vi "Write to Module.vi"(8 "error in (no error)":errorcluster, 9 "Data":u16, 10 "Module":enum16{"LAI", "LDO", "Control"}(ring), 11 "Modbus in":refnum<class "Modbus.lvclass">) -> (0 "error out":errorcluster, 3 "Modbus out":refnum<class "Modbus.lvclass">)   [LabVIEW 2020, in "Modbus.lvlib" / "Modbus.lvclass"]
uses:
  Modbus.lvclass
  Modbus.lvclass/Modbus.ctl
  <vilib>/NI Modbus.llb/MB Serial Master Query Write Multiple Registers (poly).vi
panel:
  in  "Register":u16
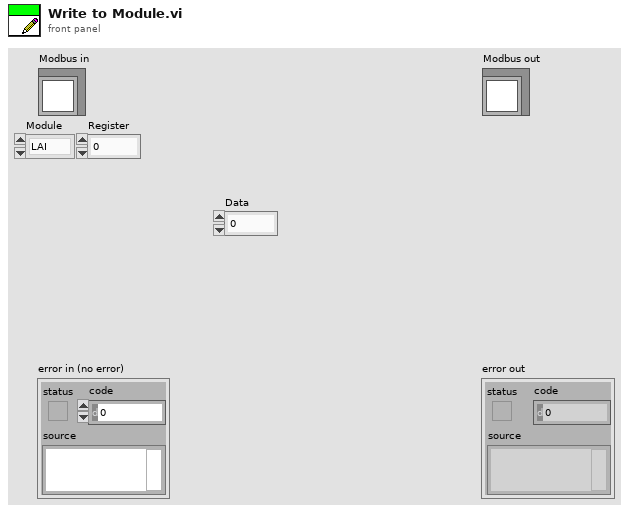
[diagram p1: front panel]
types:
  T1 = cluster{"Mode":enum16{"RTU", "ASCII"}, "Slave Address":u8}
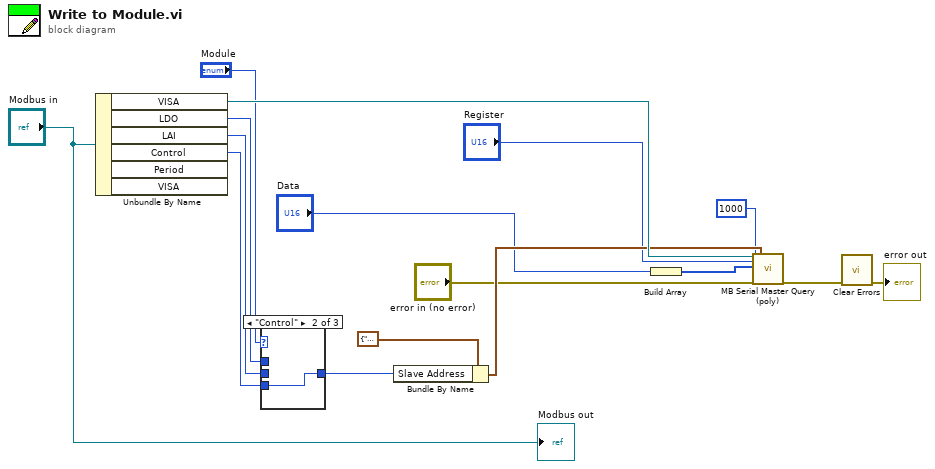
[diagram p0: block diagram]
diagram:
  n1 = Unbundle By Name("Modbus in") -> ("VISA"=w16:refnum<visa-resource-name>, "LDO"=w15:u16, "LAI"=w14:u16, "Control"=w13:u16)  [unwired: 2 out]
  n2 = case shown="\"Control\"" "Module" {
    tunnel: w15 -> [_ _ w19]
    tunnel: w14 -> [w17 _ _]
    tunnel: [w17 w18 w19] -> w5
    tunnel: w13 -> [_ w18 _]
    frame "LAI", Default {
    }
    frame "Control" {
    }
    frame "LDO" {
    }
  }
  n3 = Bundle By Name(cluster=T1 {"Mode"=enum."RTU", "Slave Address"=0} ("Serial Parameters"), "Slave Address"=w5) -> (w11:T1)
  n4 = Build Array("Data") -> (w2:u16[])
  n5 = call-poly <vilib>:"MB Serial Master Query (poly).vi"("VISA resource name"=w16, "Starting Address"="Register", "Registers"=w2, "Timeout"=u32 1000, "error in"="error in (no error)", "Serial Parameters"=w11) -> ("error out"=w9:errorcluster)  [unwired: 11 in, 2 out]
  n6 = call <vilib>:"Clear Errors.vi"("error in (no error)"=w9) -> ("error out"=→"error out":errorcluster)  [unwired: 5 in, 1 out]
  "Modbus out" <- "Modbus in"
